vi "Construct.vi"(7 "timing channel first index":i32, 8 "error in":errorcluster, 9 "biu configuration":T1, 10 "id":string, 11 "execution unit":refnum<class "Execution Unit.lvclass">) -> (0 "error out":errorcluster, 3 "execution unit out":refnum<class "Execution Unit.lvclass">)   [LabVIEW 2020, in "AIM MIL-STD-1553 Engine.lvlib" / "Implementation.lvlib" / "Execution Unit.lvclass"]
uses:
  Execution Unit.lvclass
  Execution Unit.lvclass/Execution Unit.ctl
  Shared/BIU Configuration.ctl
  Shared/Message Definition.ctl
  Shared/Terminal Endpoint.ctl
  Shared/Address.ctl
  Shared/Parameter Definition.ctl
  Shared/Message Type.ctl
  Shared/Major Frame Definition.ctl
  Shared/Minor Frame Definition.ctl
  Shared/Acyclic Frame Definition.ctl
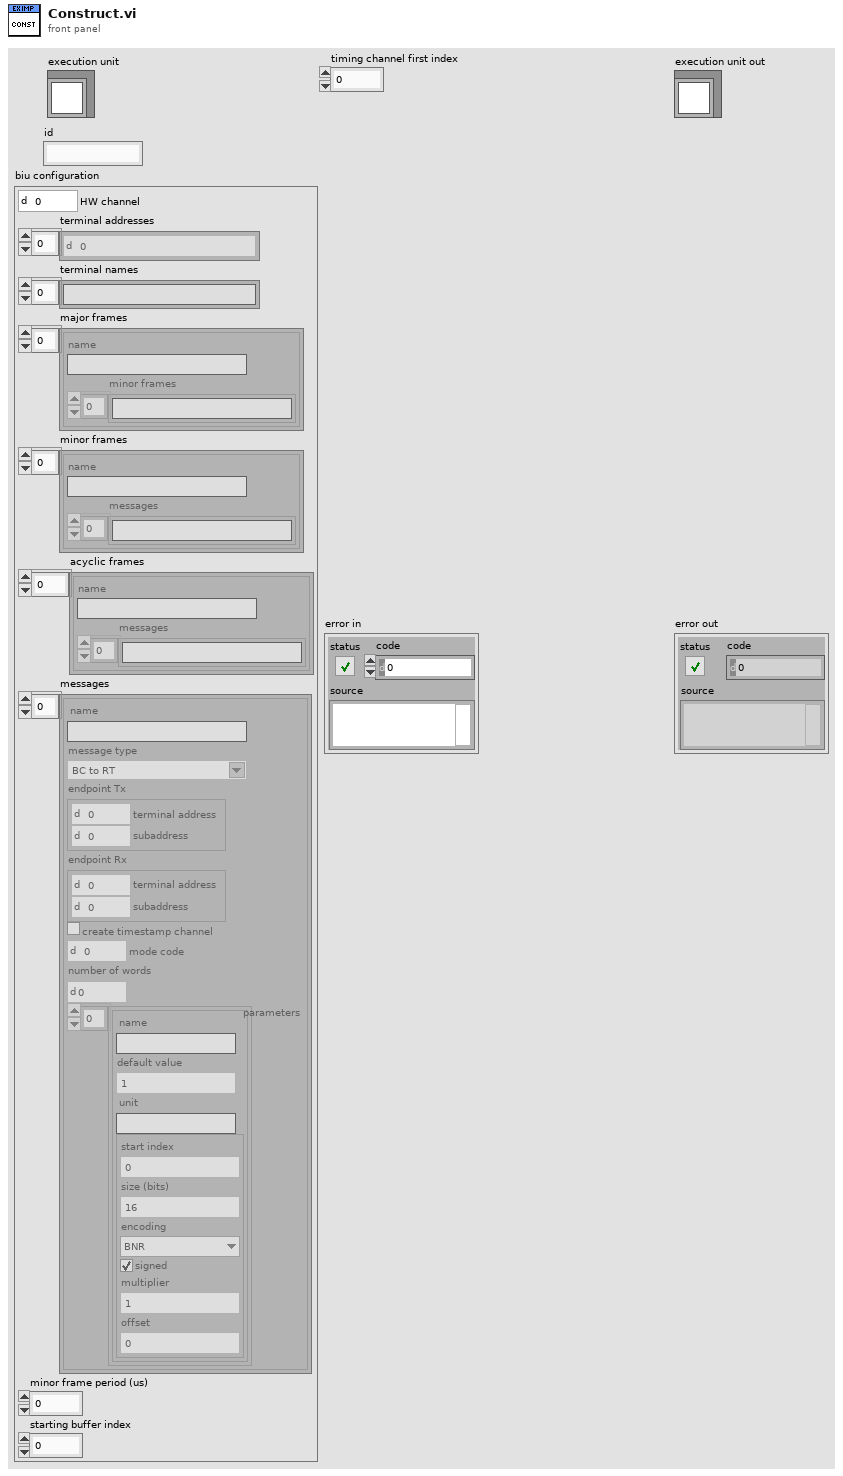
[diagram p1: front panel]
types:
  T1 = typedef "BIU Configuration.ctl" = cluster{"HW channel":u16, "terminal addresses":T2[], "terminal names":string[], "major frames":T3[], "minor frames":T4[], "acyclic frames":T5[], "messages":T6[], "minor frame period (us)":i32, "starting buffer index":u16}
  T2 = typedef "Address.ctl" = u16
  T3 = typedef "Major Frame Definition.ctl" = cluster{"name":string, "minor frames":string[]}
  T4 = typedef "Minor Frame Definition.ctl" = cluster{"name":string, "messages":string[]}
  T5 = typedef "Acyclic Frame Definition.ctl" = cluster{"name":string, "messages":string[]}
  T6 = typedef "Message Definition.ctl" = cluster{"name":string, "message type":T7, "endpoint Tx":T8, "endpoint Rx":T8, "create timestamp channel":bool, "mode code":u16, "number of words":u16, "parameters":cluster{"name":string, "default value":dbl, "unit":string, "parameter definition":T9}[]}
  T7 = typedef "Message Type.ctl" = string
  T8 = typedef "Terminal Endpoint.ctl" = cluster{"terminal address":T2, "subaddress":T2}
  T9 = typedef "Parameter Definition.ctl" = cluster{"start index":i32, "size (bits)":i32, "encoding":enum16{"BNR", "BCD", "Discrete"}, "signed":bool, "multiplier":dbl, "offset":dbl}
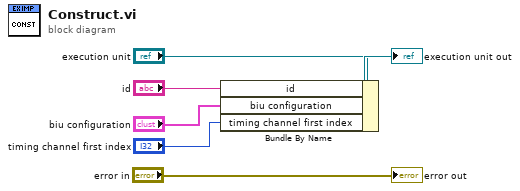
[diagram p0: block diagram]
diagram:
  n1 = Bundle By Name(cluster="execution unit", "id"="id", "biu configuration"="biu configuration", "timing channel first index"="timing channel first index") -> (→"execution unit out":refnum<class "Execution Unit.lvclass">)
  "error out" <- "error in"
